vi "ClsTakeReference.vi"(8 "error in (no error)":errorcluster, 10 "take white and dark reference?":bool, 11 "Connection Out in":u32) -> (0 "error out":errorcluster)   [LabVIEW 2015]
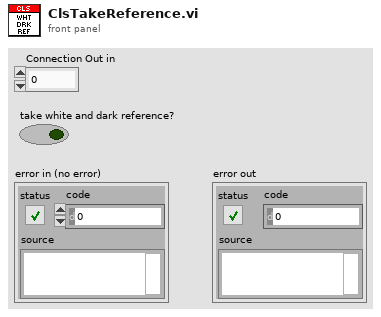
[diagram p1: front panel]
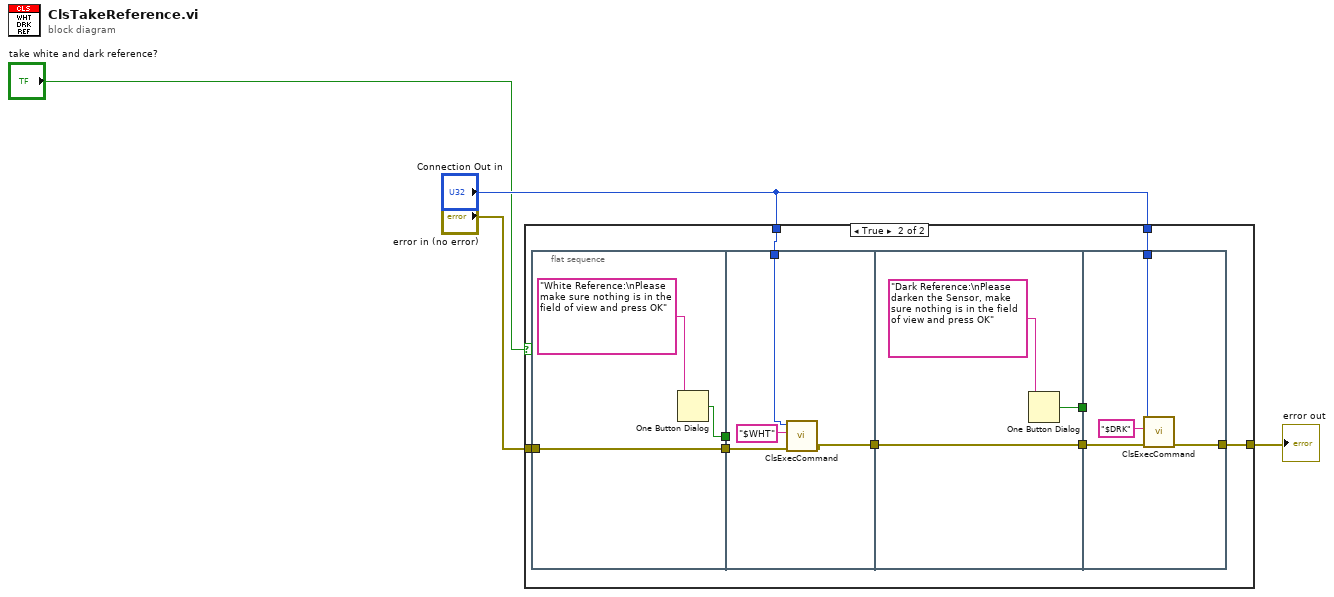
[diagram p0: block diagram]
diagram:
  n1 = case shown="True" "take white and dark reference?" {
    tunnel: "error in (no error)" -> [w5 w12]
    tunnel: "Connection Out in" -> [_ w11]
    tunnel: "Connection Out in" -> [_ w9]
    tunnel: [w5 w6] -> w3
    frame False {
    }
    frame True {
      n2 = flat-sequence {
        tunnel: [w16] -> w14
        tunnel: [w15] -> w13
        tunnel: w12 -> [w15]
        tunnel: w14 -> [_]
        tunnel: w13 -> [w20]
        tunnel: w11 -> [w19]
        tunnel: [w18] -> w8
        tunnel: [w23] -> w10
        tunnel: w8 -> [w22]
        tunnel: [w22] -> w7
        tunnel: w10 -> [_]
        tunnel: w9 -> [w28]
        tunnel: w7 -> [w26]
        tunnel: [w25] -> w6
        frame #0 {
          n3 = One Button Dialog(message="White Reference:\nPlease make sure nothing is in the field of view and press OK") -> (true=w16:bool)  [unwired: 1 in]
        }
        frame #1 {
          n4 = call "ClsExecCommand.vi"("error in (no error)"=w20, "Command In"="$WHT", "Connection In"=w19) -> ("error out"=w18:errorcluster)  [unwired: 6 in, 2 out]
        }
        frame #2 {
          n5 = One Button Dialog(message="Dark Reference:\nPlease darken the Sensor, make sure nothing is in the field of view and press OK") -> (true=w23:bool)  [unwired: 1 in]
        }
        frame #3 {
          n6 = call "ClsExecCommand.vi"("error in (no error)"=w26, "Command In"="$DRK", "Connection In"=w28) -> ("error out"=w25:errorcluster)  [unwired: 6 in, 2 out]
        }
      }
    }
  }
  "error out" <- w3
